vi "Z-Scan Intensity EXP.vi"(5 "APD":tag="/Dev2/PFI0", 7 "Counter":tag="Dev2/ctr0", 8 "error in":errorcluster, 10 "Scan parameters":T1={"Number of Steps"=100, "Start (mm)"=10.0, "10 (mm)"=90.0}, 11 "RS232 settings":cluster{"Portnumber":i32, "Baudrate":u16}={"Portnumber"=12, "Baudrate"=5} {"Portnumber" items=["COM1", "COM2", "COM3", "COM4", "COM5", "COM6", "COM7", "COM8", "COM9", "COM10", "COM11", "COM12", "COM13", "COM14", "COM15", "COM16", "COM17", "COM18", "COM19", "COM20", "COM21", "COM22", "COM23", "COM24", "COM25", "COM26", "COM27", "COM28", "COM29", "COM30"]; "Baudrate" items=["9600", "14400", "19200", "38400", "57600", "115200"]}) -> (0 "error out":errorcluster, 2 "Max Intensity":u32, 3 "XY Graph":cluster{"Y":dbl[], "Y":dbl[]}[](graph))   [LabVIEW 2011]
uses:
  <vilib>/DAQmx/read.llb/DAQmx Read (Counter U32 1Chan 1Samp).vi
  <vilib>/DAQmx/create/channels.llb/DAQmx Create Channel (CI-Count Edges).vi
  <vilib>/DAQmx/miscellaneous.llb/DAQmx Fill In Error Info.vi
  Program Files/National Instruments/LabVIEW 2011/resource/objmgr/daqmx.rc
panel:
  in  "stop 2":bool
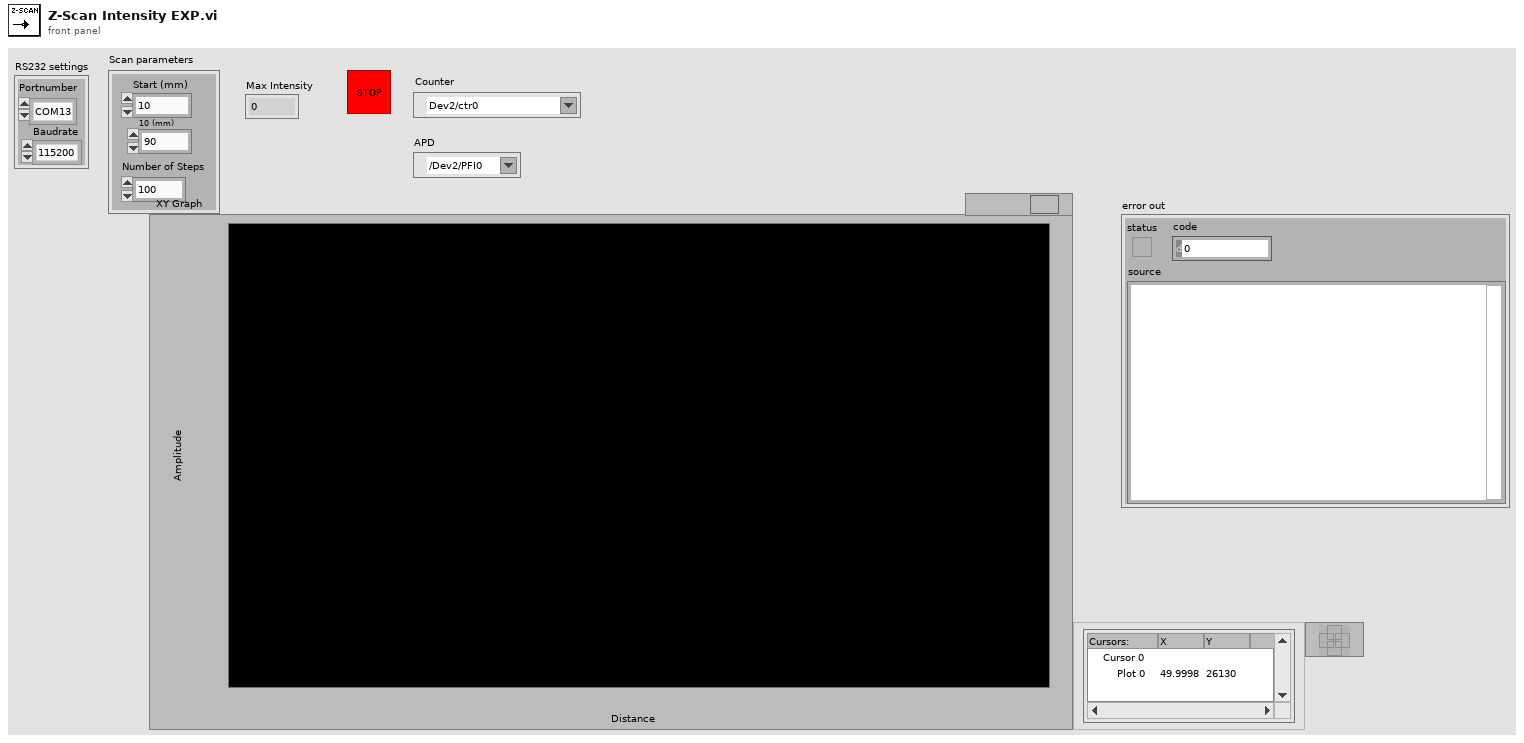
[diagram p1: front panel]
types:
  T1 = cluster{"Number of Steps":i32, "Start (mm)":dbl, "10 (mm)":dbl}
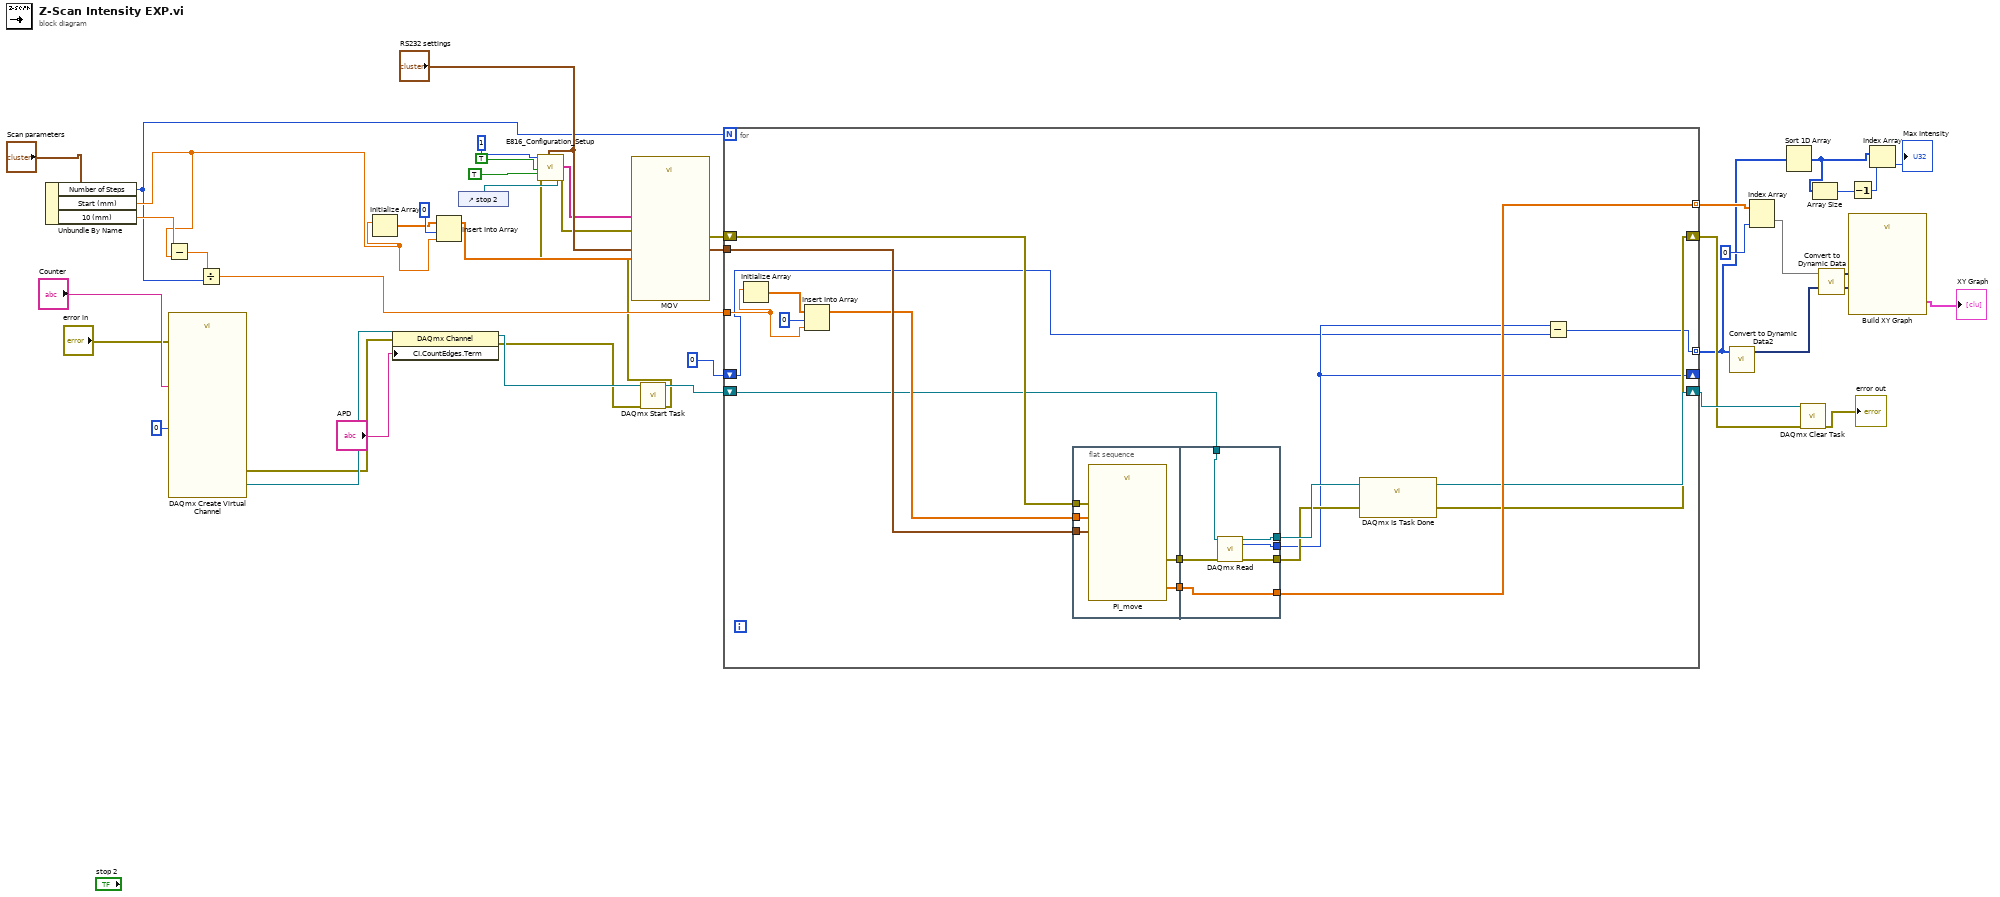
[diagram p0: block diagram]
diagram:
  n1 = Unbundle By Name("Scan parameters") -> ("Number of Steps"=w12:i32, "Start (mm)"=w13:dbl, "10 (mm)"=w14:dbl)
  n2 = Subtract(x=w14, y=w13) -> (x-y=w33:dbl)
  n3 = call-poly <vilib>:"DAQmx Create Virtual Channel.vi"("initial count"=u32 0, "counter"="Counter", "error in"="error in") -> ("task out"=w42:refnum<k21>, "error out"=w41:errorcluster)  [unwired: 5 in, 6 out]
  n4 = Divide(x=w33, y=w12) -> (x/y=w32:dbl)
  n5 = Initialize Array(w13) -> (w29:dbl[])  [unwired: 1 in]
  n6 = property class="DAQmx Channel"(reference=w42, error in=w41, "CI.CountEdges.Term"="APD") -> (reference out=w8:refnum<k21>, error out=w7:errorcluster)
  n7 = Insert Into Array(array=w29, index=0, new element=w13) -> (w28:dbl[])
  n8 = control-ref of="stop 2"() -> (w26:refnum<vi>)
  n9 = call <vilib>:"DAQmx Start Task.vi"("task/channels in"=w8, "error in"=w7) -> ("task out"=w39:refnum<k21>, "error out"=w21:errorcluster)  [unwired: 12 in]
  n10 = call "E816_Configuration_Setup.vi"("System no."=1, "All axes?"=TRUE, "Change servo \nstatus to ON?"=TRUE ("Use dialog to define\nconnected stages?"), "error in"=w21, "RS232 settings"="RS232 settings", "Stop refnum"=w26) -> ("Conn. Axes"=w22:string[], "error out"=w20:errorcluster)  [unwired: 10 in, 2 out]
  n11 = call "MOV.vi"("Axes to move"=w22, "Position values"=w28, "error in"=w20) -> ("error out"=w31:errorcluster)  [unwired: 16 in]
  n12 = for {
    N: w12 -> [_]
    tunnel: "RS232 settings" -> [w59]
    tunnel: w32 -> [w53]
    shift-right: [w46] -> w18
    shift-left: w31 -> [w55]
    tunnel: [w54] -> w37 mode=indexing
    shift-right: [w47] -> w19
    shift-left: w39 -> [w50]
    tunnel: [w43] -> w6 mode=indexing
    shift-right: [w45] -> _
    shift-left: u32 0 ("data") -> [w44]
    n13 = Initialize Array(w53) -> (w56:dbl[])  [unwired: 1 in]
    n14 = Insert Into Array(array=w56, index=0, new element=w53) -> (w57:dbl[])
    n15 = flat-sequence {
      tunnel: w59 -> [w64]
      tunnel: w57 -> [w63]
      tunnel: w55 -> [w62]
      tunnel: [w61] -> w52
      tunnel: [w60] -> w51
      tunnel: [w70] -> w54
      tunnel: w52 -> [w70]
      tunnel: w51 -> [w68]
      tunnel: w50 -> [w65]
      tunnel: [w69] -> w49
      tunnel: [w67] -> w48
      tunnel: [w66] -> w45
      frame #0 {
        n16 = call "PI_move.vi"("RS232 settings"=w64, "Position values"=w63, "error in"=w62) -> ("Position"=w61:dbl[], "error out"=w60:errorcluster)  [unwired: 14 in, 1 out]
      }
      frame #1 {
        n17 = call-poly <vilib>:"DAQmx Read.vi"("task/channels in"=w65, "error in"=w68) -> ("task out"=w69:refnum<k21>, "data"=w66:u32, "error out"=w67:errorcluster)  [unwired: 2 in, 9 out]
      }
    }
    n18 = call <vilib>:"DAQmx Is Task Done.vi"("task/channels in"=w49, "error in"=w48) -> ("task out"=w47:refnum<k21>, "error out"=w46:errorcluster)  [unwired: 12 out]
    n19 = Subtract(x=w45, y=w44) -> (x-y=w43:u32)
  }
  n20 = call "Convert to Dynamic Data2"("Array"=w6) -> ("Dynamic Data Type"=w38:dynamicdata)  [unwired: 3 in]
  n21 = Index Array(array=w37, index (col)=0 ("index (row)")) -> (element=w36:dbl[])  [unwired: 1 in]
  n22 = Sort 1D Array(array=w6) -> (sorted array=w3:u32[])
  n23 = call <vilib>:"DAQmx Clear Task.vi"("task in"=w19, "error in"=w18) -> ("error out"=→"error out":errorcluster)  [unwired: 13 in]
  n24 = Array Size(array=w3) -> (size(s)=w4:i32)
  n25 = call "Convert to Dynamic Data"("Array"=w36) -> ("Dynamic Data Type"=w35:dynamicdata)  [unwired: 3 in]
  n26 = call "Build XY Graph"("Y Input"=w38, "X Input"=w35) -> ("XY Graph"=→"XY Graph":cluster{"Y":dbl[], "Y":dbl[]}[])  [unwired: 3 in, 6 out]
  n27 = Decrement(x=w4) -> (x-1=w2:i32)
  n28 = Index Array(array=w3, index=w2) -> (element=→"Max Intensity":u32)
